vi "Log_Comando.vi"(1 "Erro":bool, 2 "string do Comando":string, 3 "string da resposta":string, 4 "String":string, 5 "Erro de Resposta":bool, 6 "Erro Recebido":bool) -> ()   [LabVIEW 2018]
uses:
  Global_Telescopio.vi
panel:
  out "before substring":string
  out "Comando":string
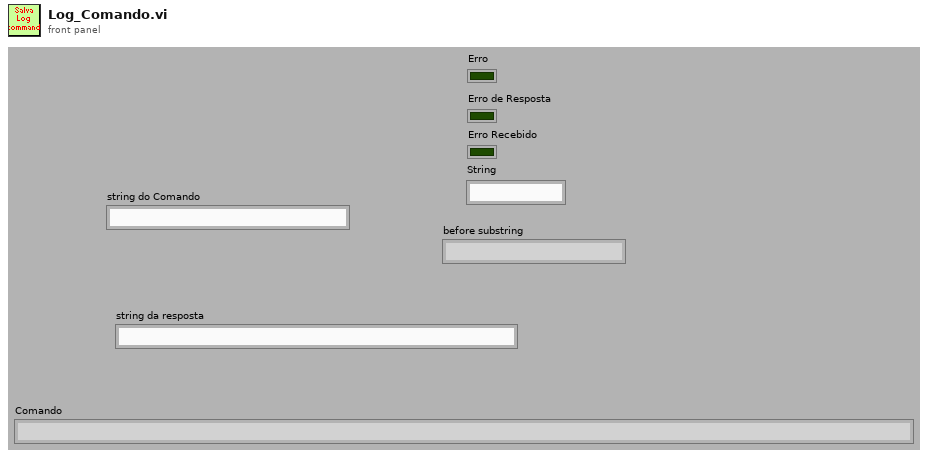
[diagram p1: front panel]
types:
  T1 = enum16{"open", "open or create", "create or replace", "create"}
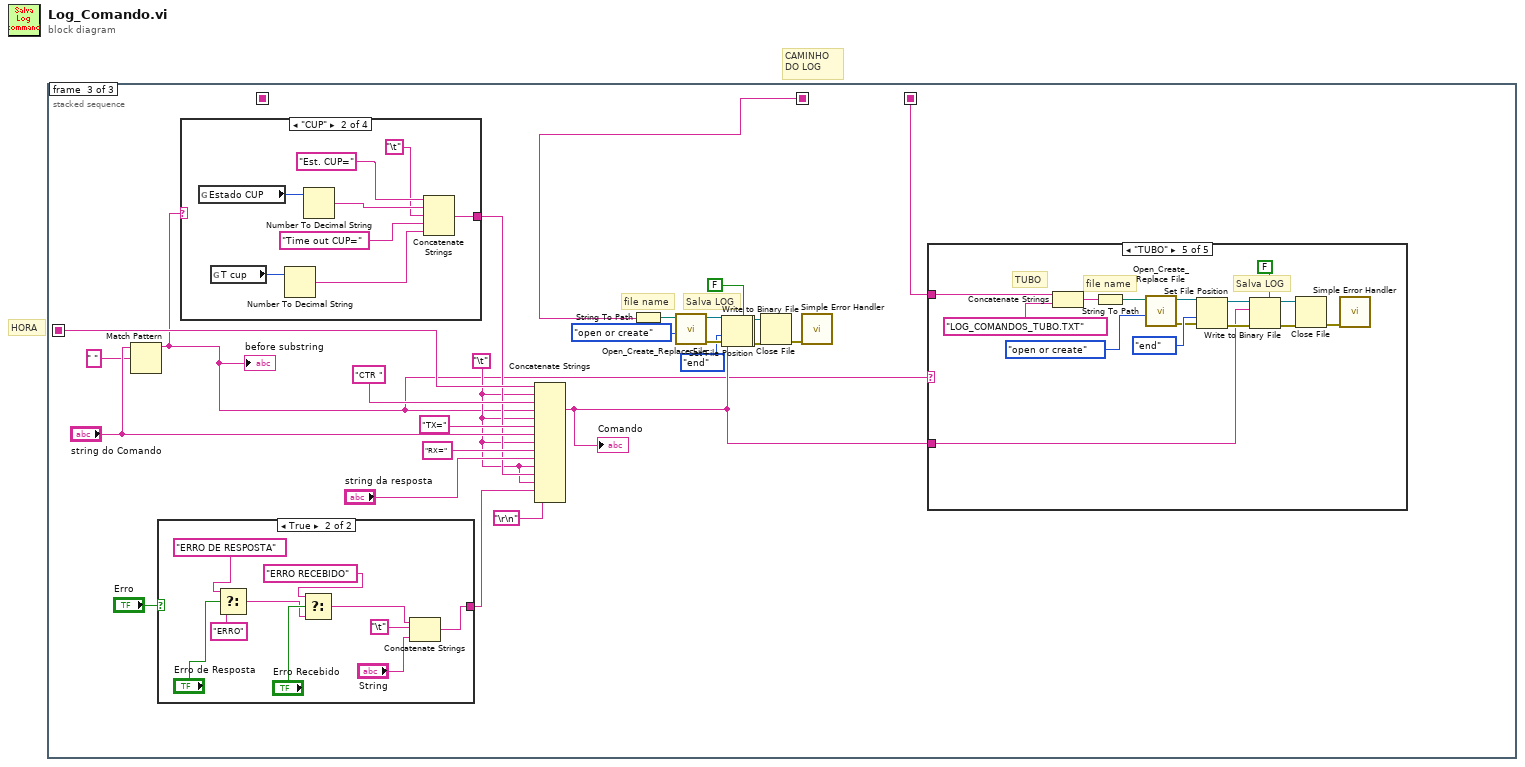
[diagram p0: block diagram]
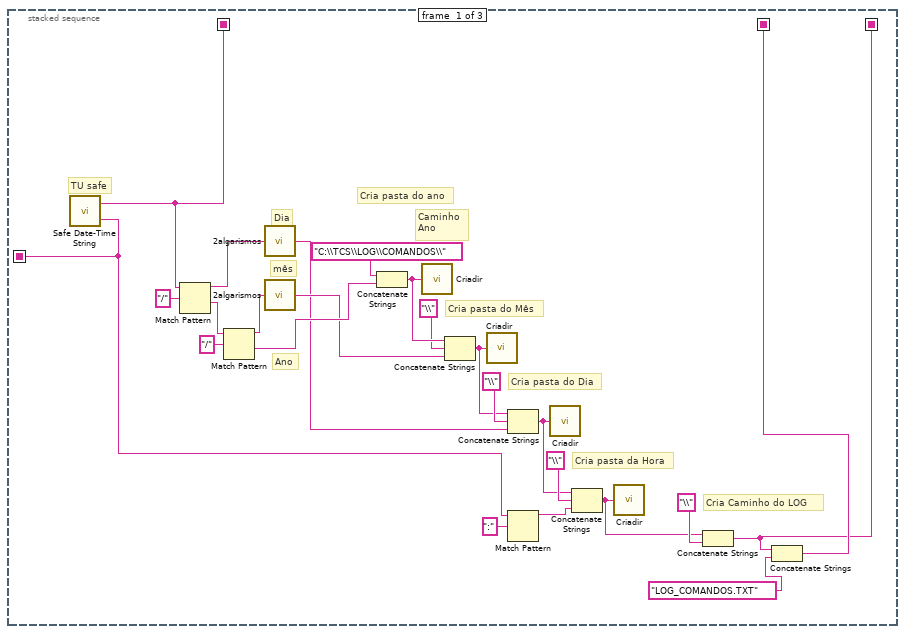
[diagram p2: hidden frame]
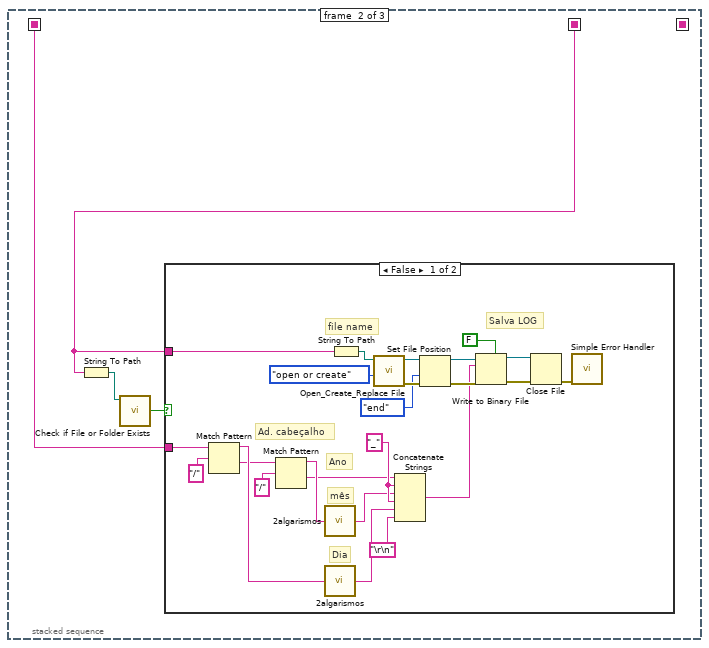
[diagram p3: hidden frame]
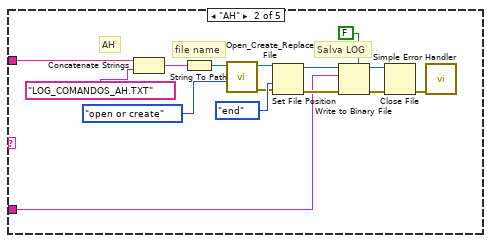
[diagram p6: hidden frame]
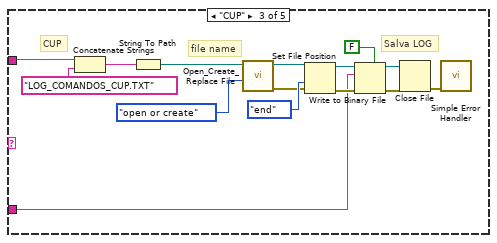
[diagram p7: hidden frame]
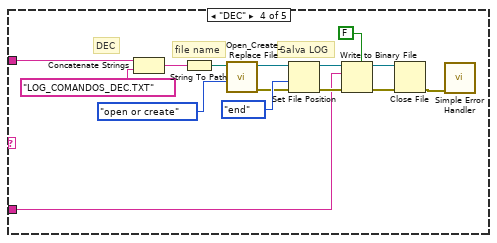
[diagram p8: hidden frame]
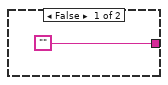
[diagram p9: hidden frame]
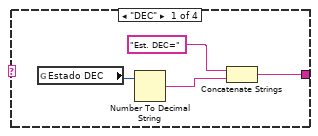
[diagram p10: hidden frame]
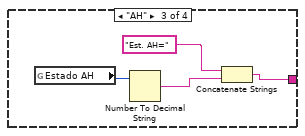
[diagram p11: hidden frame]
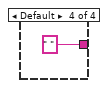
[diagram p12: hidden frame]
diagram:
  # "CAMINHO\nDO LOG"
  # "HORA"
  n1 = stacked-sequence {
    seq-local: [w4 _ _] -> [_ w27 w56]
    seq-local: [w1 _ _] -> [_ _ w78]
    seq-local: [w2 _ _] -> [_ w28 _]
    seq-local: [w3 _ _] -> [_ _ w54]
    frame #0 {
      # "TU safe"
      # "Cria pasta da Hora"
      # "Cria Caminho do LOG"
      # "Cria pasta do Dia"
      # "Cria pasta do Mês"
      # "Caminho\nAno"
      # "Ano"
      # "mês"
      # "Dia"
      # "Cria pasta do ano"
      n2 = call "Safe Date-Time String.vi"() -> ("Safe time string"=w1:string, "Safe date string"=w2:string)  [unwired: 3 in]
      n3 = Match Pattern(string=w2, regular expression="/") -> (before substring=w21:string, after substring=w22:string)  [unwired: 1 in, 2 out]
      n4 = Match Pattern(string=w22, regular expression="/") -> (before substring=w20:string, after substring=w18:string)  [unwired: 1 in, 2 out]
      n5 = call "2algarismos.vi"("entrada"=w21) -> ("saida"=w12:string)
      n6 = call "2algarismos.vi"("entrada"=w20) -> ("saida"=w15:string)
      n7 = Concatenate Strings("C:\\TCS\\LOG\\COMANDOS\\" ("SOMENTE DIRETORIO"), w18) -> (w17:string)
      n8 = call "Criadir.vi"("SOMENTE DIRETORIO"=w17) -> ()  [unwired: 2 out]
      n9 = Concatenate Strings(w17, "\\" ("regular expression"), w15) -> (w13:string)
      n10 = call "Criadir.vi"("SOMENTE DIRETORIO"=w13) -> ()  [unwired: 2 out]
      n11 = Concatenate Strings(w13, "\\" ("regular expression"), w12) -> (w9:string)
      n12 = Match Pattern(string=w1, regular expression=":") -> (before substring=w7:string)  [unwired: 1 in, 3 out]
      n13 = call "Criadir.vi"("SOMENTE DIRETORIO"=w9) -> ()  [unwired: 2 out]
      n14 = Concatenate Strings(w9, "\\" ("regular expression"), w7) -> (w6:string)
      n15 = call "Criadir.vi"("SOMENTE DIRETORIO"=w6) -> ()  [unwired: 2 out]
      n16 = Concatenate Strings(w6, "\\" ("regular expression")) -> (w3:string)
      n17 = Concatenate Strings(w3, "LOG_COMANDOS.TXT" ("regular expression")) -> (w4:string)
    }
    frame #1 {
      n18 = String To Path(string=w27) -> (path=w26:path)
      n19 = call <vilib>:"Check if File or Folder Exists.vi"("path"=w26) -> ("file or folder exists?"=w25:bool)  [unwired: 8 in, 2 out]
      n20 = case shown="False" w25 {
        tunnel: w27 -> [w41 _]
        tunnel: w28 -> [w31 _]
        frame False {
          w39 = "_"
          # "Ad. cabeçalho"
          # "Ano"
          # "mês"
          # "Dia"
          # "Salva LOG"
          # "file name"
          n21 = Match Pattern(string=w31, regular expression="/") -> (before substring=w40:string, after substring=w37:string)  [unwired: 1 in, 2 out]
          n22 = Match Pattern(string=w37, regular expression="/") -> (before substring=w36:string, after substring=w35:string)  [unwired: 1 in, 2 out]
          n23 = call "2algarismos.vi"("entrada"=w36) -> ("saida"=w34:string)
          n24 = call "2algarismos.vi"("entrada"=w40) -> ("saida"=w33:string)
          n25 = String To Path(string=w41) -> (path=w45:path)
          n26 = call <vilib>:"Open_Create_Replace File.vi"("function (open:0)"=T1."open or create", "file path"=w45) -> ("error out"=w48:errorcluster, "refnum"=w51:refnum<file>)  [unwired: 6 in, 2 out]
          n27 = Concatenate Strings(w35, w39, w34, w39, w33, "\r\n") -> (w32:string)
          n28 = Set File Position(refnum=w51, from (0:start)=enum16{"start", "end", "current"}."end" ("pos mode (0:2)"), error in=w48) -> (refnum out=w44:refnum<file>, error out=w43:errorcluster)  [unwired: 1 in]
          n29 = Write to Binary File(file (use dialog)=w44, data=w32, error in=w43, 5:FALSE ("prepend array or string size? (T)")) -> (refnum out=w50:refnum<file>, error out=w49:errorcluster)  [unwired: 2 in, 1 out]
          n30 = Close File(refnum=w50, error in=w49) -> (error out=w52:errorcluster)  [unwired: 1 out]
          n31 = call <vilib>:"Simple Error Handler.vi"("error in (no error)"=w52) -> ()  [unwired: 4 in, 5 out]
        }
        frame True {
        }
      }
    }
    frame #2 {
      w59 = "\t"
      # "Salva LOG"
      # "file name"
      n32 = Match Pattern(string="string do Comando", regular expression=" ") -> (before substring=w53:string)  [unwired: 1 in, 3 out]
      "before substring" <- w53
      n33 = case shown="True" "Erro" {
        tunnel: ["" w141] -> w58
        frame False {
        }
        frame True {
          n34 = Select(t="ERRO DE RESPOSTA", s="Erro de Resposta", f="ERRO") -> (s? t:f=w146:string)
          n35 = Select(t="ERRO RECEBIDO", s="Erro Recebido", f=w146) -> (s? t:f=w144:string)
          n36 = Concatenate Strings(w144, "\t", "String") -> (w141:string)
        }
      }
      n37 = case shown="\"CUP\"" w53 {
        tunnel: [w151 w155 w163 " "] -> w61
        frame "DEC" {
          n38 = global read "Global_Telescopio.vi" "Estado DEC"() -> (w154:i32)
          n39 = Number To Decimal String(number=w154) -> (decimal integer string=w152:string)  [unwired: 1 in]
          n40 = Concatenate Strings("Est. DEC=", w152) -> (w151:string)
        }
        frame "CUP" {
          n41 = global read "Global_Telescopio.vi" "Estado CUP"() -> (w160:i32)
          n42 = global read "Global_Telescopio.vi" "T cup"() -> (w158:u32)
          n43 = Number To Decimal String(number=w158) -> (decimal integer string=w156:string)  [unwired: 1 in]
          n44 = Number To Decimal String(number=w160) -> (decimal integer string=w161:string)  [unwired: 1 in]
          n45 = Concatenate Strings("Est. CUP=", w161, "\t", "Time out CUP=", w156) -> (w155:string)
        }
        frame "AH" {
          n46 = global read "Global_Telescopio.vi" "Estado AH"() -> (w166:i32)
          n47 = Number To Decimal String(number=w166) -> (decimal integer string=w164:string)  [unwired: 1 in]
          n48 = Concatenate Strings("Est. AH=", w164) -> (w163:string)
        }
        frame Default {
        }
      }
      n49 = Concatenate Strings(w78, w59, "CTR ", w53, w59, "TX=", "string do Comando", w59, "RX=", "string da resposta", w59, w61, w59, w58, "\r\n") -> (w55:string)
      "Comando" <- w55
      n50 = String To Path(string=w56) -> (path=w70:path)
      n51 = call <vilib>:"Open_Create_Replace File.vi"("function (open:0)"=T1."open or create", "file path"=w70) -> ("error out"=w73:errorcluster, "refnum"=w76:refnum<file>)  [unwired: 6 in, 2 out]
      n52 = Set File Position(refnum=w76, from (0:start)=enum16{"start", "end", "current"}."end" ("pos mode (0:2)"), error in=w73) -> (refnum out=w66:refnum<file>, error out=w65:errorcluster)  [unwired: 1 in]
      n53 = Write to Binary File(file (use dialog)=w66, data=w55, error in=w65, 5:FALSE ("prepend array or string size? (T)")) -> (refnum out=w75:refnum<file>, error out=w74:errorcluster)  [unwired: 2 in, 1 out]
      n54 = Close File(refnum=w75, error in=w74) -> (error out=w77:errorcluster)  [unwired: 1 out]
      n55 = call <vilib>:"Simple Error Handler.vi"("error in (no error)"=w77) -> ()  [unwired: 4 in, 5 out]
      n56 = case shown="\"TUBO\"" w53 {
        tunnel: w54 -> [_ w94 w109 w124 w139]
        tunnel: w55 -> [_ w80 w95 w110 w125]
        frame "False", Default {
        }
        frame "AH" {
          # "Salva LOG"
          # "file name"
          # "AH"
          n57 = Concatenate Strings(w94, "LOG_COMANDOS_AH.TXT" ("regular expression")) -> (w81:string)
          n58 = String To Path(string=w81) -> (path=w89:path)
          n59 = call <vilib>:"Open_Create_Replace File.vi"("function (open:0)"=T1."open or create", "file path"=w89) -> ("error out"=w86:errorcluster, "refnum"=w83:refnum<file>)  [unwired: 6 in, 2 out]
          n60 = Set File Position(refnum=w83, from (0:start)=enum16{"start", "end", "current"}."end" ("pos mode (0:2)"), error in=w86) -> (refnum out=w90:refnum<file>, error out=w91:errorcluster)  [unwired: 1 in]
          n61 = Write to Binary File(file (use dialog)=w90, data=w80, error in=w91, 5:FALSE ("prepend array or string size? (T)")) -> (refnum out=w84:refnum<file>, error out=w85:errorcluster)  [unwired: 2 in, 1 out]
          n62 = Close File(refnum=w84, error in=w85) -> (error out=w82:errorcluster)  [unwired: 1 out]
          n63 = call <vilib>:"Simple Error Handler.vi"("error in (no error)"=w82) -> ()  [unwired: 4 in, 5 out]
        }
        frame "CUP" {
          # "Salva LOG"
          # "file name"
          # "CUP"
          n64 = Concatenate Strings(w109, "LOG_COMANDOS_CUP.TXT" ("regular expression")) -> (w96:string)
          n65 = String To Path(string=w96) -> (path=w104:path)
          n66 = call <vilib>:"Open_Create_Replace File.vi"("function (open:0)"=T1."open or create", "file path"=w104) -> ("error out"=w101:errorcluster, "refnum"=w98:refnum<file>)  [unwired: 6 in, 2 out]
          n67 = Set File Position(refnum=w98, from (0:start)=enum16{"start", "end", "current"}."end" ("pos mode (0:2)"), error in=w101) -> (refnum out=w105:refnum<file>, error out=w106:errorcluster)  [unwired: 1 in]
          n68 = Write to Binary File(file (use dialog)=w105, data=w95, error in=w106, 5:FALSE ("prepend array or string size? (T)")) -> (refnum out=w99:refnum<file>, error out=w100:errorcluster)  [unwired: 2 in, 1 out]
          n69 = Close File(refnum=w99, error in=w100) -> (error out=w97:errorcluster)  [unwired: 1 out]
          n70 = call <vilib>:"Simple Error Handler.vi"("error in (no error)"=w97) -> ()  [unwired: 4 in, 5 out]
        }
        frame "DEC" {
          # "DEC"
          # "Salva LOG"
          # "file name"
          n71 = Concatenate Strings(w124, "LOG_COMANDOS_DEC.TXT" ("regular expression")) -> (w111:string)
          n72 = String To Path(string=w111) -> (path=w119:path)
          n73 = call <vilib>:"Open_Create_Replace File.vi"("function (open:0)"=T1."open or create", "file path"=w119) -> ("error out"=w116:errorcluster, "refnum"=w113:refnum<file>)  [unwired: 6 in, 2 out]
          n74 = Set File Position(refnum=w113, from (0:start)=enum16{"start", "end", "current"}."end" ("pos mode (0:2)"), error in=w116) -> (refnum out=w120:refnum<file>, error out=w121:errorcluster)  [unwired: 1 in]
          n75 = Write to Binary File(file (use dialog)=w120, data=w110, error in=w121, 5:FALSE ("prepend array or string size? (T)")) -> (refnum out=w114:refnum<file>, error out=w115:errorcluster)  [unwired: 2 in, 1 out]
          n76 = Close File(refnum=w114, error in=w115) -> (error out=w112:errorcluster)  [unwired: 1 out]
          n77 = call <vilib>:"Simple Error Handler.vi"("error in (no error)"=w112) -> ()  [unwired: 4 in, 5 out]
        }
        frame "TUBO" {
          # "TUBO"
          # "Salva LOG"
          # "file name"
          n78 = Concatenate Strings(w139, "LOG_COMANDOS_TUBO.TXT" ("regular expression")) -> (w126:string)
          n79 = String To Path(string=w126) -> (path=w134:path)
          n80 = call <vilib>:"Open_Create_Replace File.vi"("function (open:0)"=T1."open or create", "file path"=w134) -> ("error out"=w131:errorcluster, "refnum"=w128:refnum<file>)  [unwired: 6 in, 2 out]
          n81 = Set File Position(refnum=w128, from (0:start)=enum16{"start", "end", "current"}."end" ("pos mode (0:2)"), error in=w131) -> (refnum out=w135:refnum<file>, error out=w136:errorcluster)  [unwired: 1 in]
          n82 = Write to Binary File(file (use dialog)=w135, data=w125, error in=w136, 5:FALSE ("prepend array or string size? (T)")) -> (refnum out=w129:refnum<file>, error out=w130:errorcluster)  [unwired: 2 in, 1 out]
          n83 = Close File(refnum=w129, error in=w130) -> (error out=w127:errorcluster)  [unwired: 1 out]
          n84 = call <vilib>:"Simple Error Handler.vi"("error in (no error)"=w127) -> ()  [unwired: 4 in, 5 out]
        }
      }
    }
  }
